vi "Write LIDAR Range Data.vi"(8 "Mask":bool[](array[boolean]), 9 "Range Data":dbl[](array[numeric]), 10 "Direction (deg)":dbl[](array[numeric]), 11 "Magnitude  (mm)":dbl[](array[numeric])) -> (1 "Range Data":dbl[](array[numeric]))   [LabVIEW 2011]
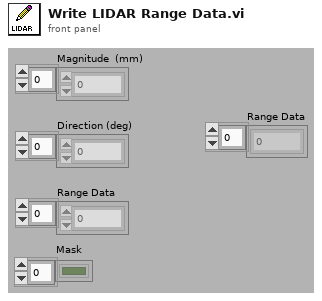
[diagram p1: front panel]
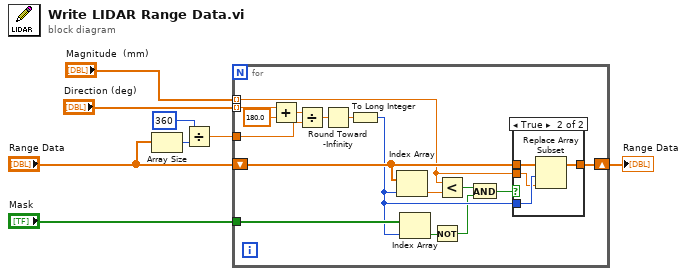
[diagram p0: block diagram]
diagram:
  n1 = Array Size(array="Range Data") -> (size(s)=w5:i32)
  n2 = Divide(x=360, y=w5) -> (x/y=w8:dbl)
  n3 = for {
    shift-right: [w14] -> w4
    shift-left: "Range Data" -> [w16]
    tunnel: "Magnitude  (mm)" -> [w15] mode=indexing
    tunnel: "Direction (deg)" -> [w24] mode=indexing
    tunnel: w8 -> [w21]
    tunnel: "Mask" -> [w13]
    n4 = Add(x=w24, y=180.0) -> (x+y=w22:dbl)
    n5 = Divide(x=w22, y=w21) -> (x/y=w20:dbl)
    n6 = Round Toward -Infinity(1:w20) -> (0:w19:dbl)
    n7 = To Long Integer(number=w19) -> (32bit integer=w12:i32)
    n8 = Index Array(array=w16, index=w12) -> (element=w18:dbl)
    n9 = Index Array(array=w13, index=w12) -> (element=w10:bool)
    n10 = Not(x=w10) -> (.not. x?=w9:bool)
    n11 = Less?(x=w15, y=w18) -> (x < y?=w17:bool)
    n12 = And(x=w17, y=w9) -> (x .and. y?=w11:bool)
    n13 = case shown="True" w11 {
      tunnel: w12 -> [_ w28]
      tunnel: w16 -> [w25 w29]
      tunnel: w15 -> [_ w27]
      tunnel: [w25 w26] -> w14
      frame False {
      }
      frame True {
        n14 = Replace Array Subset(array=w29, new element=w27, index=w28) -> (w26:dbl[])
      }
    }
  }
  "Range Data" <- w4
